vi "O2 to Lambda.vi"(1 "O2 %":sgl) -> (0 "Lambda":dbl)   [LabVIEW 2014]
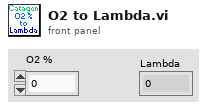
[diagram p1: front panel]
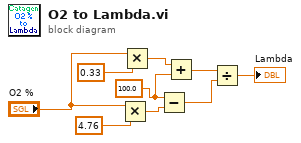
[diagram p0: block diagram]
diagram:
  w3 = 100.0 ("x")
  n1 = Multiply(x="O2 %", y=4.76) -> (x*y=w8:dbl)
  n2 = Multiply(x="O2 %", y=0.33) -> (x*y=w4:dbl)
  n3 = Subtract(x=w3, y=w8) -> (x-y=w6:dbl)
  n4 = Add(x=w4, y=w3) -> (x+y=w2:dbl)
  n5 = Divide(x=w2, y=w6) -> (x/y=→"Lambda":dbl)
